vi "選擇難易度.vi"() -> (0 "HARD":bool, 1 "EASY":bool)   [LabVIEW 2014]
panel:
  in  "OK Button 3":bool
  in  "OK Button 2":bool
  in  "OK Button":bool
  # "歡迎來到青蛙歷險記\n請選擇難易度"
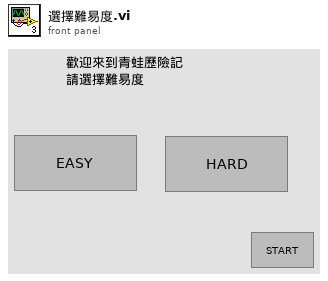
[diagram p1: front panel]
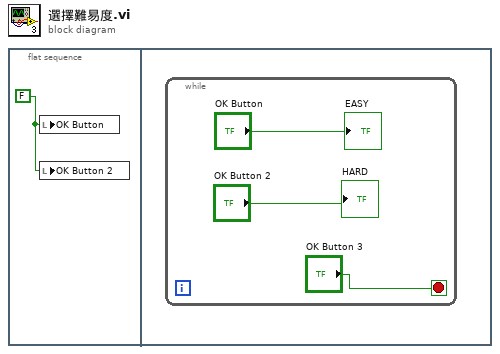
[diagram p0: block diagram]
diagram:
  n1 = flat-sequence {
    frame #0 {
      w1 = FALSE ("OK Button")
      n2 = local write "OK Button"(w1) -> ()
      n3 = local write "OK Button 2"(w1) -> ()
    }
    frame #1 {
      n4 = while {
        stop <- "OK Button 3" stop-if-true
        "EASY" <- "OK Button"
        "HARD" <- "OK Button 2"
      }
    }
  }
